vi "Create.vi"(7 "Direction":T1, 8 "error in (no error)":errorcluster, 9 "Custom Config Data":u8[](array[numeric]), 10 "Name":string, 11 "CIFTag in":refnum<class "CIF_NIChn_Fifo_DAQ.lvclass">) -> (0 "error out":errorcluster, 3 "CIFTag out":refnum<class "CIF_NIChn_Fifo_DAQ.lvclass">)   [LabVIEW 2021, in "CIF_NIChn_Fifo_DAQ.lvclass"]
uses:
  CIF_NIChn_Fifo_DAQ.lvclass
  D:/dev/CIF-LVCore/src/Channels/CIFChannels/CIFChannels.lvclass
  D:/dev/CIF-LVCore/src/Channels/CIF_NIChn/NIChn/CIF_NIChn.lvclass
  CIFChannels/Typedef/Direction.ctl
  CIFChannels/Typedef/Disconnect Behavior.ctl
  CIF_NIChn_Fifo_DAQ.lvclass/CIF_NIChn_Fifo_DAQ.ctl
  ChannelCommon/CIFFIFO/CIFfifo.lvclass/CIFfifo.ctl
  CIFChannels/CIFChannels.lvclass/CIFChannels.ctl
  ChannelCommon/typedef/Datatype Waveform.ctl
  CIFChannels/Typedef/Channel State.ctl
  NIChn/CIF_NIChn.lvclass/CIF_NIChn.ctl
  c6f1aac1-fdda-4143-8087-f9e7d57e6170.vi
  05c6e502-0377-480c-a15d-085597602460.vi
  CIFChannels/Accessors/Write Channel State.vi
  NIChn/Accessors/Write CIF Channel.vi
  CIFChannels/SubVIs/Get Type from Class.vi
  CIFChannels/Accessors/Write Type.vi
  CIFChannels/Accessors/Write Channel Class.vi
  CIFChannels/Accessors/Write Direction.vi
  CIFChannels/Accessors/Write Disconnect Behavior.vi
  CIFChannels/Accessors/Write Name.vi
  CIFChannels/Accessors/Write Custom Config Data.vi
  <vilib>/CIFChannels/SubVIs/Add Error.vi
  c6f1aac1-fdda-4143-8087-f9e7d57e6170.vi/c28b0ead-42ad-4072-80a2-aca7f2bd7ce3.vi
  <vilib>/CIFChannels/SubVIs/CIFServices Fill In Error Info Ex.vi
  <vilib>/CIFChannels/SubVIs/Get dll Path.vi
  c6f1aac1-fdda-4143-8087-f9e7d57e6170.vi/259f1102-a6f3-45ef-83a9-e8a266e5a7b9.vi
  05c6e502-0377-480c-a15d-085597602460.vi/c28b0ead-42ad-4072-80a2-aca7f2bd7ce3.vi
  ChannelCommon/Utilities/Unflatten FIFO Config.vi
  ChannelCommon/CIFFIFO/Accessors/Write Header.vi
  ChannelCommon/CIFFIFO/Accessors/Write Flags.vi
  ChannelCommon/CIFFIFO/Accessors/Write ClockID.vi
  <vilib>/CIFChannels/SubVIs/Append Error Location.vi
  ChannelCommon/Utilities/Expand FIFO Flags.vi
  <vilib>/Utility/LVClass/Get LV Class Name.vi
  CIFChannels/CIFChannels.lvclass
  ChannelCommon/CIFFIFO/CIFfifo.lvclass
  ChannelCommon/ChannelCommon.lvlib
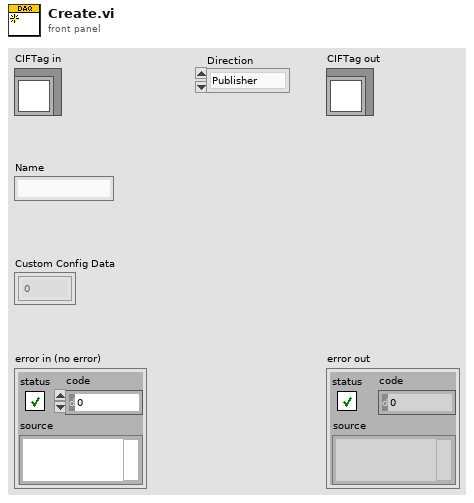
[diagram p1: front panel]
types:
  T1 = typedef "CIFChannels.lvclass/Direction.ctl" = enum16{"Publisher", "Subscriber"}
  T2 = typedef "CIFChannels.lvclass/Disconnect Behavior.ctl" = enum16{"Default value", "Last value", "Error with default"}
  T3 = typedef "ChannelCommon.lvlib/Datatype Waveform.ctl" = cluster{"measurement":dbl[], "dT":dbl, "Timestamp":u64, "Read Lock":bool}
  T4 = typedef "CIFChannels.lvclass/Channel State.ctl" = enum16{"Creating", "Disconnected", "Connecting", "Connected", "Destroyed"}
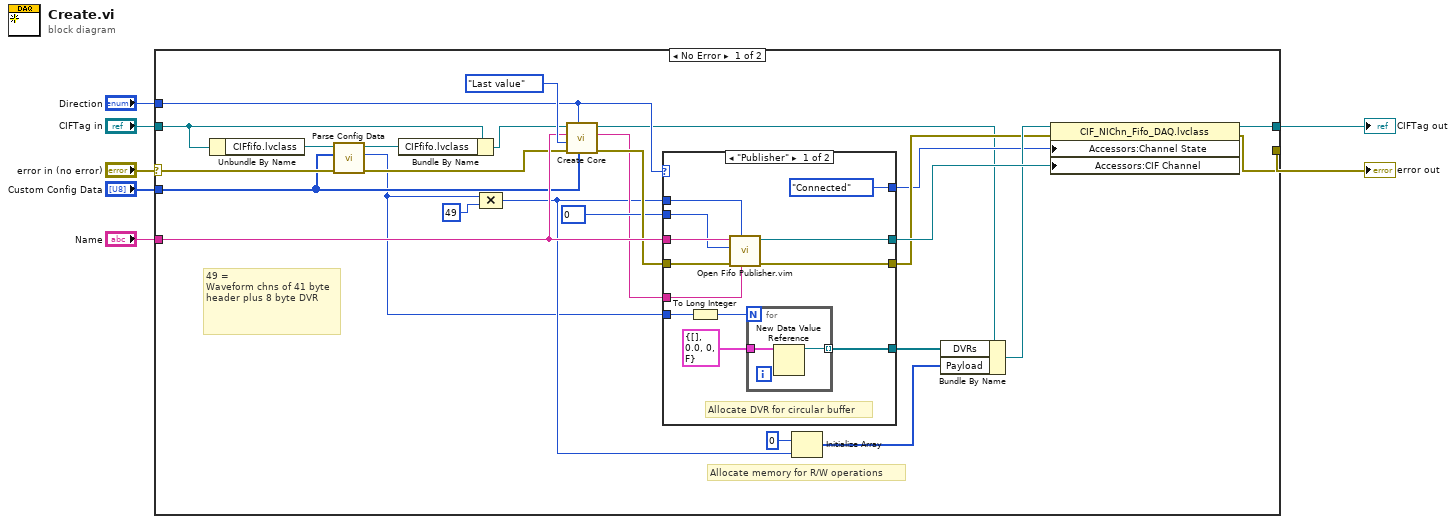
[diagram p0: block diagram]
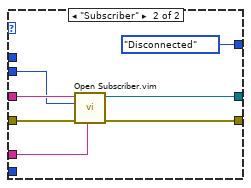
[diagram p2: hidden frame]
diagram:
  n1 = case shown="No Error" "error in (no error)" {
    selector: "error in (no error)" -> [w16 w56]
    tunnel: [w32 w56] -> w6
    tunnel: [w26 w55] -> w4
    tunnel: "CIFTag in" -> [w19 w55]
    tunnel: "Name" -> [w31 _]
    tunnel: "Direction" -> [w25 _]
    tunnel: "Custom Config Data" -> [w14 _]
    frame No Error {
      # "49 =\nWaveform chns of 41 byte header plus 8 byte DVR"
      # "Allocate memory for R/W operations"
      n2 = Unbundle By Name(w19) -> ("CIFfifo.lvclass"=w18:refnum<class "CIFfifo.lvclass">)
      n3 = call "Parse Config Data.vi"("error in (no error)"=w16, "Custom Config Data"=w14, "CIFfifo in"=w18) -> ("error out"=w15:errorcluster, "Depth"=w9:u64, "CIFfifo out"=w17:refnum<class "CIFfifo.lvclass">)  [unwired: 6 in]
      n4 = Bundle By Name(cluster=w19, "CIFfifo.lvclass"=w17) -> (w21:refnum<class "CIF_NIChn_Fifo_DAQ.lvclass">)
      n5 = Compound Arithmetic op=MULTIPLY(w9, u64 49 ("y")) -> (w11:u64)
      n6 = call "Create Core.vi"("Custom Config Data"=w14, "Direction"=w25, "error in (no error)"=w15, "Disconnect Behavior"=Disconnect_Behavior."Last value", "Name"=w31, "CIFChannels in"=w21) -> ("error out"=w30:errorcluster, "Channel Type"=w20:string, "CIFChannels out"=w23:refnum<class "CIF_NIChn_Fifo_DAQ.lvclass">)  [unwired: 3 in]
      n7 = case shown="\"Publisher\"" w25 {
        tunnel: w31 -> [w45 w53]
        tunnel: w30 -> [w44 w52]
        tunnel: [w40 w48] -> w29
        tunnel: [w41 w49] -> w27
        tunnel: w20 -> [w43 w51]
        tunnel: [Channel_State."Connected" ("Channel State") Channel_State."Disconnected" ("Channel State")] -> w24
        tunnel: u8 0 -> [w39 w50]
        tunnel: w11 -> [w38 _]
        tunnel: w9 -> [w35 _]
        tunnel: [w37 _] -> w8
        frame "Publisher" {
          # "Allocate DVR for circular buffer"
          n8 = To Long Integer(number=w35) -> (32bit integer=w34:i32)
          n9 = call "Open Fifo Publisher.vim"("Channel Type Description"=w43, "depth"=w38, "error in"=w44, "Input Type"=w39, "Channel Name"=w45) -> ("error out"=w41:errorcluster, "CIF Channel"=w40:refnum<k21>)  [unwired: 5 in]
          n10 = for {
            N: w34 -> [_]
            tunnel: T3 {"measurement"=[], "dT"=0.0, "Timestamp"=0, "Read Lock"=FALSE} ("Waveform Datatype") -> [w47]
            tunnel: [w46] -> w37 mode=indexing
            n11 = New Data Value Reference(data value=w47) -> (data value reference=w46:refnum<data-value>)  [unwired: 1 in, 1 out]
          }
        }
        frame "Subscriber" {
          n12 = call "Open Subscriber.vim"("Channel Type Description"=w51, "error in"=w52, "Input Type"=w50, "Channel Name"=w53) -> ("error out"=w49:errorcluster, "CIF Channel"=w48:refnum<k21>)  [unwired: 6 in]
        }
      }
      n13 = Initialize Array(u8 0 ("Numeric"), w11) -> (w10:u8[])
      n14 = Bundle By Name(cluster=w23, "DVRs"=w8, "Payload"=w10) -> (w28:refnum<class "CIF_NIChn_Fifo_DAQ.lvclass">)
      n15 = property class="CIF_NIChn_Fifo_DAQ.lvclass"(reference=w28, error in=w27, "Accessors:Channel State"=w24, "Accessors:CIF Channel"=w29) -> (reference out=w26:refnum<class "CIF_NIChn_Fifo_DAQ.lvclass">, error out=w32:errorcluster)
    }
    frame Error {
    }
  }
  "error out" <- w6
  "CIFTag out" <- w4
